vi "CANOpen_Get PDO Name from Channel.vi"(11 "PDO Channel":u8) -> (3 "PDO Channel Name":string)   [LabVIEW 2021, in "CANOpen Addon System Explorer.lvlib"]
uses:
  CANOpen Addon System Explorer.lvlib
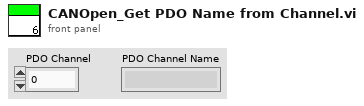
[diagram p1: front panel]
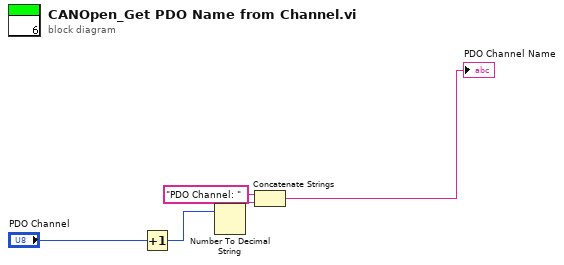
[diagram p0: block diagram]
diagram:
  n1 = Increment(x="PDO Channel") -> (x+1=w5:u8)
  n2 = Number To Decimal String(number=w5) -> (decimal integer string=w2:string)  [unwired: 1 in]
  n3 = Concatenate Strings("PDO Channel: " ("string"), w2) -> (→"PDO Channel Name":string)
